vi "Set Index.vi"(8 "error in (no error)":errorcluster, 10 "Index":i32, 11 "Boolean_1D in":refnum<class "Boolean_1D.lvclass">) -> (0 "error out":errorcluster, 3 "Boolean_1D out":refnum<class "Boolean_1D.lvclass">)   [LabVIEW 2021, in "Boolean_1D.lvclass"]
uses:
  Boolean_1D.lvclass
  Boolean_1D.lvclass/Boolean_1D.ctl
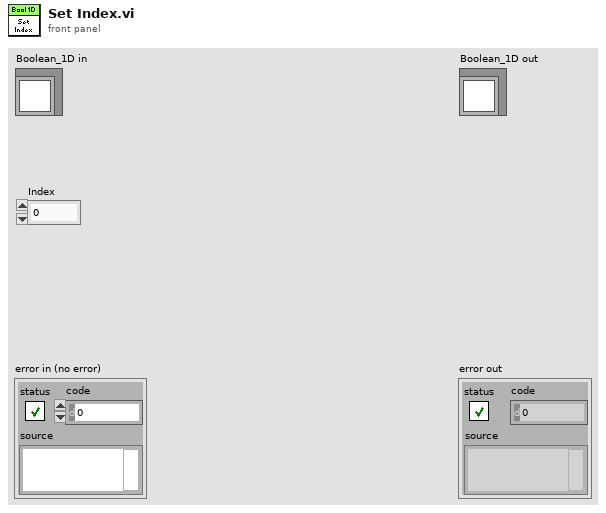
[diagram p1: front panel]
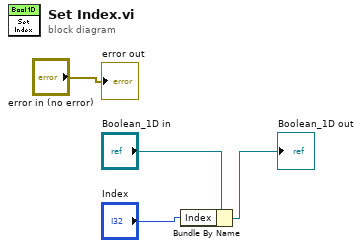
[diagram p0: block diagram]
diagram:
  n1 = Bundle By Name(cluster="Boolean_1D in", "Index"="Index") -> (→"Boolean_1D out":refnum<class "Boolean_1D.lvclass">)
  "error out" <- "error in (no error)"
